vi "Periodic Tasks.vi"(8 "error in":errorcluster) -> ()   [LabVIEW 2012]
doc: "This VI runs in parallel to other tasks. It can contain as many user-defined periodic loops as you need. These can carry out PID or other sorts of timed response."
uses:
  <vilib>/Rock Robotics/WPI/Relay/WPI_RelayValue.ctl
  <vilib>/Rock Robotics/SystemInterfaces/Utilities/FPGA_UtilitiesLED Source.ctl
  <vilib>/Rock Robotics/SystemInterfaces/Utilities/FPGA_UtilitiesLED State.ctl
  <vilib>/Rock Robotics/WPI/Joystick/WPI_JoystickGetSetRefNum.vi
  Robot Global Data.vi
  <vilib>/Rock Robotics/WPI/Solenoid/WPI_SolenoidSetEnum.vi
  <vilib>/Rock Robotics/WPI/Compressor/WPI_CompressorGetSetRefNum.vi
panel:
  out "Ball Shooter motor speed":dbl
  out "s? t:f 4":dbl
  out "s? t:f 3":dbl
  out "s? t:f 2":dbl
  out "s? t:f":dbl
  out "Number of Balls in the Hopper":dbl
  in  "Starting Number Balls":i32=2
  out "Total Number of shots made":i16
  out "Hopper State":bool
  out "Ball in Hopper":bool
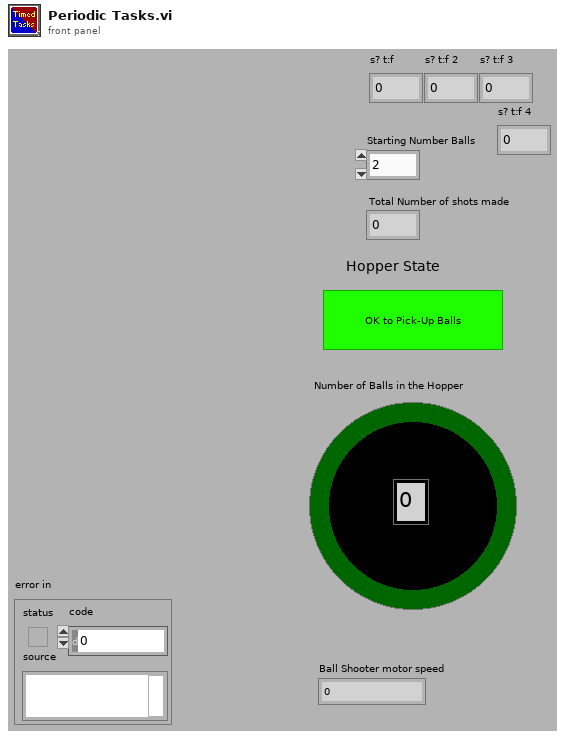
[diagram p1: front panel]
types:
  T1 = typedef "WPI_MotorControlDeviceRef.ctl" = cluster{"DeviceStatus":errorcluster, "Type":enum16{"PWM", "CAN"}, "PWM":cluster{"Digital Module":T2, "PWM Channel":T3, "DeadBand":T4}, "CAN":cluster{"Device Number":u8, "Control Mode":T5, "Semaphore":T6, "Max Vout":dbl}, "Invert":bool, "TransformRef":T7, "InvTransformRef":T7}
  T2 = typedef "FPGA_TypedefDigitalModule.ctl" = enum16{"Digital Module 1", "Digital Module 2"}
  T3 = typedef "FPGA_DIOPWMChannel.ctl" = enum8{"PWM 1", "PWM 2", "PWM 3", "PWM 4", "PWM 5", "PWM 6", "PWM 7", "PWM 8", "PWM 9", "PWM 10", "Invalid"}
  T4 = typedef "WPI_PWMDeadband.ctl" = cluster{"Name":string, "maxPositivePwm":i32, "minPositivePwm":i32, "centerPwm":i32, "maxNegativePwm":i32, "minNegativePwm":i32, "angularRange":u16}
  T5 = typedef "WPI_CANJaguar_ControlMode.ctl" = enum8{"Percent VBus", "Current", "Speed", "Position", "Voltage"}
  T6 = typedef "Semaphore RefNum" = refnum<k1>
  T7 = typedef "WPI_PWMTransform_ConPane.ctl" = refnum<vi>
  T8 = typedef "WPI_SolenoidDevRef.ctl" = cluster{"DevStatus":errorcluster, "Solenoid Module":T9, "Forward Solenoid Channel":T10, "Reverse Solenoid Channel":T10}
  T9 = typedef "FPGA_TypedefSolenoidModule.ctl" = enum16{"Solenoid Module 1", "Solenoid Module 2"}
  T10 = typedef "WPI_SolenoidChannel.ctl" = enum8{"Solenoid 1", "Solenoid 2", "Solenoid 3", "Solenoid 4", "Solenoid 5", "Solenoid 6", "Solenoid 7", "Solenoid 8", "Invalid"}
  T11 = typedef "WPI_JoystickDevRef.ctl" = cluster{"Device":T12}
  T12 = typedef "WPI_JoystickDeviceEnum.ctl" = enum16{"USB 1", "USB 2", "USB 3", "USB 4", "Kinect 1", "Kinect 2"}
  T13 = cluster{"MotorControlDevRef":T1, "MotorControlDevRef":T1, "MotorControlDevRef":T1, "MotorControlDevRef":T1}
  T14 = typedef "WPI_RelayValue.ctl" = enum16{"Off", "On", "Forward", "Reverse"}
  T15 = typedef "WPI_JoystickButtonState.ctl" = cluster{"Button 1":bool, "Button 2":bool, "Button 3":bool, "Button 4":bool, "Button 5":bool, "Button 6":bool, "Button 7":bool, "Button 8":bool, "Button 9":bool, "Button 10":bool, "Button 11":bool, "Button 12":bool}
  T16 = typedef "WPI_DigitalInputDevRef.ctl" = cluster{"DevStatus":errorcluster, "DIO Channel":T17, "Digital Module":T2}
  T17 = typedef "FPGA_DIOChannel.ctl" = enum8{"DIO 1", "DIO 2", "DIO 3", "DIO 4", "DIO 5", "DIO 6", "DIO 7", "DIO 8", "DIO 9", "DIO 10", "DIO 11", "DIO 12", "DIO 13", "DIO 14", "Invalid"}
  T18 = typedef "FPGA_UtilitiesLED State.ctl" = enum16{"Off", "On", "Toggle"}
  T19 = typedef "FPGA_UtilitiesLED Source.ctl" = enum16{"User LED", "FPGA LED"}
  T20 = typedef "WPI_CompressorDevRef.ctl" = cluster{"DevStatus":errorcluster, "DigitalInputDevRef":T16, "RelayDevRef":T21}
  T21 = typedef "WPI_RelayDevRef.ctl" = cluster{"DevStatus":errorcluster, "Relay Channel":T22, "Digital Module":T2, "Relay Direction":T23}
  T22 = typedef "FPGA_DIORelayChannel.ctl" = enum8{"Relay 1", "Relay 2", "Relay 3", "Relay 4", "Relay 5", "Relay 6", "Relay 7", "Relay 8", "Invalid"}
  T23 = typedef "WPI_RelayDirection.ctl" = enum16{"Both directions", "Forward only", "Reverse only"}
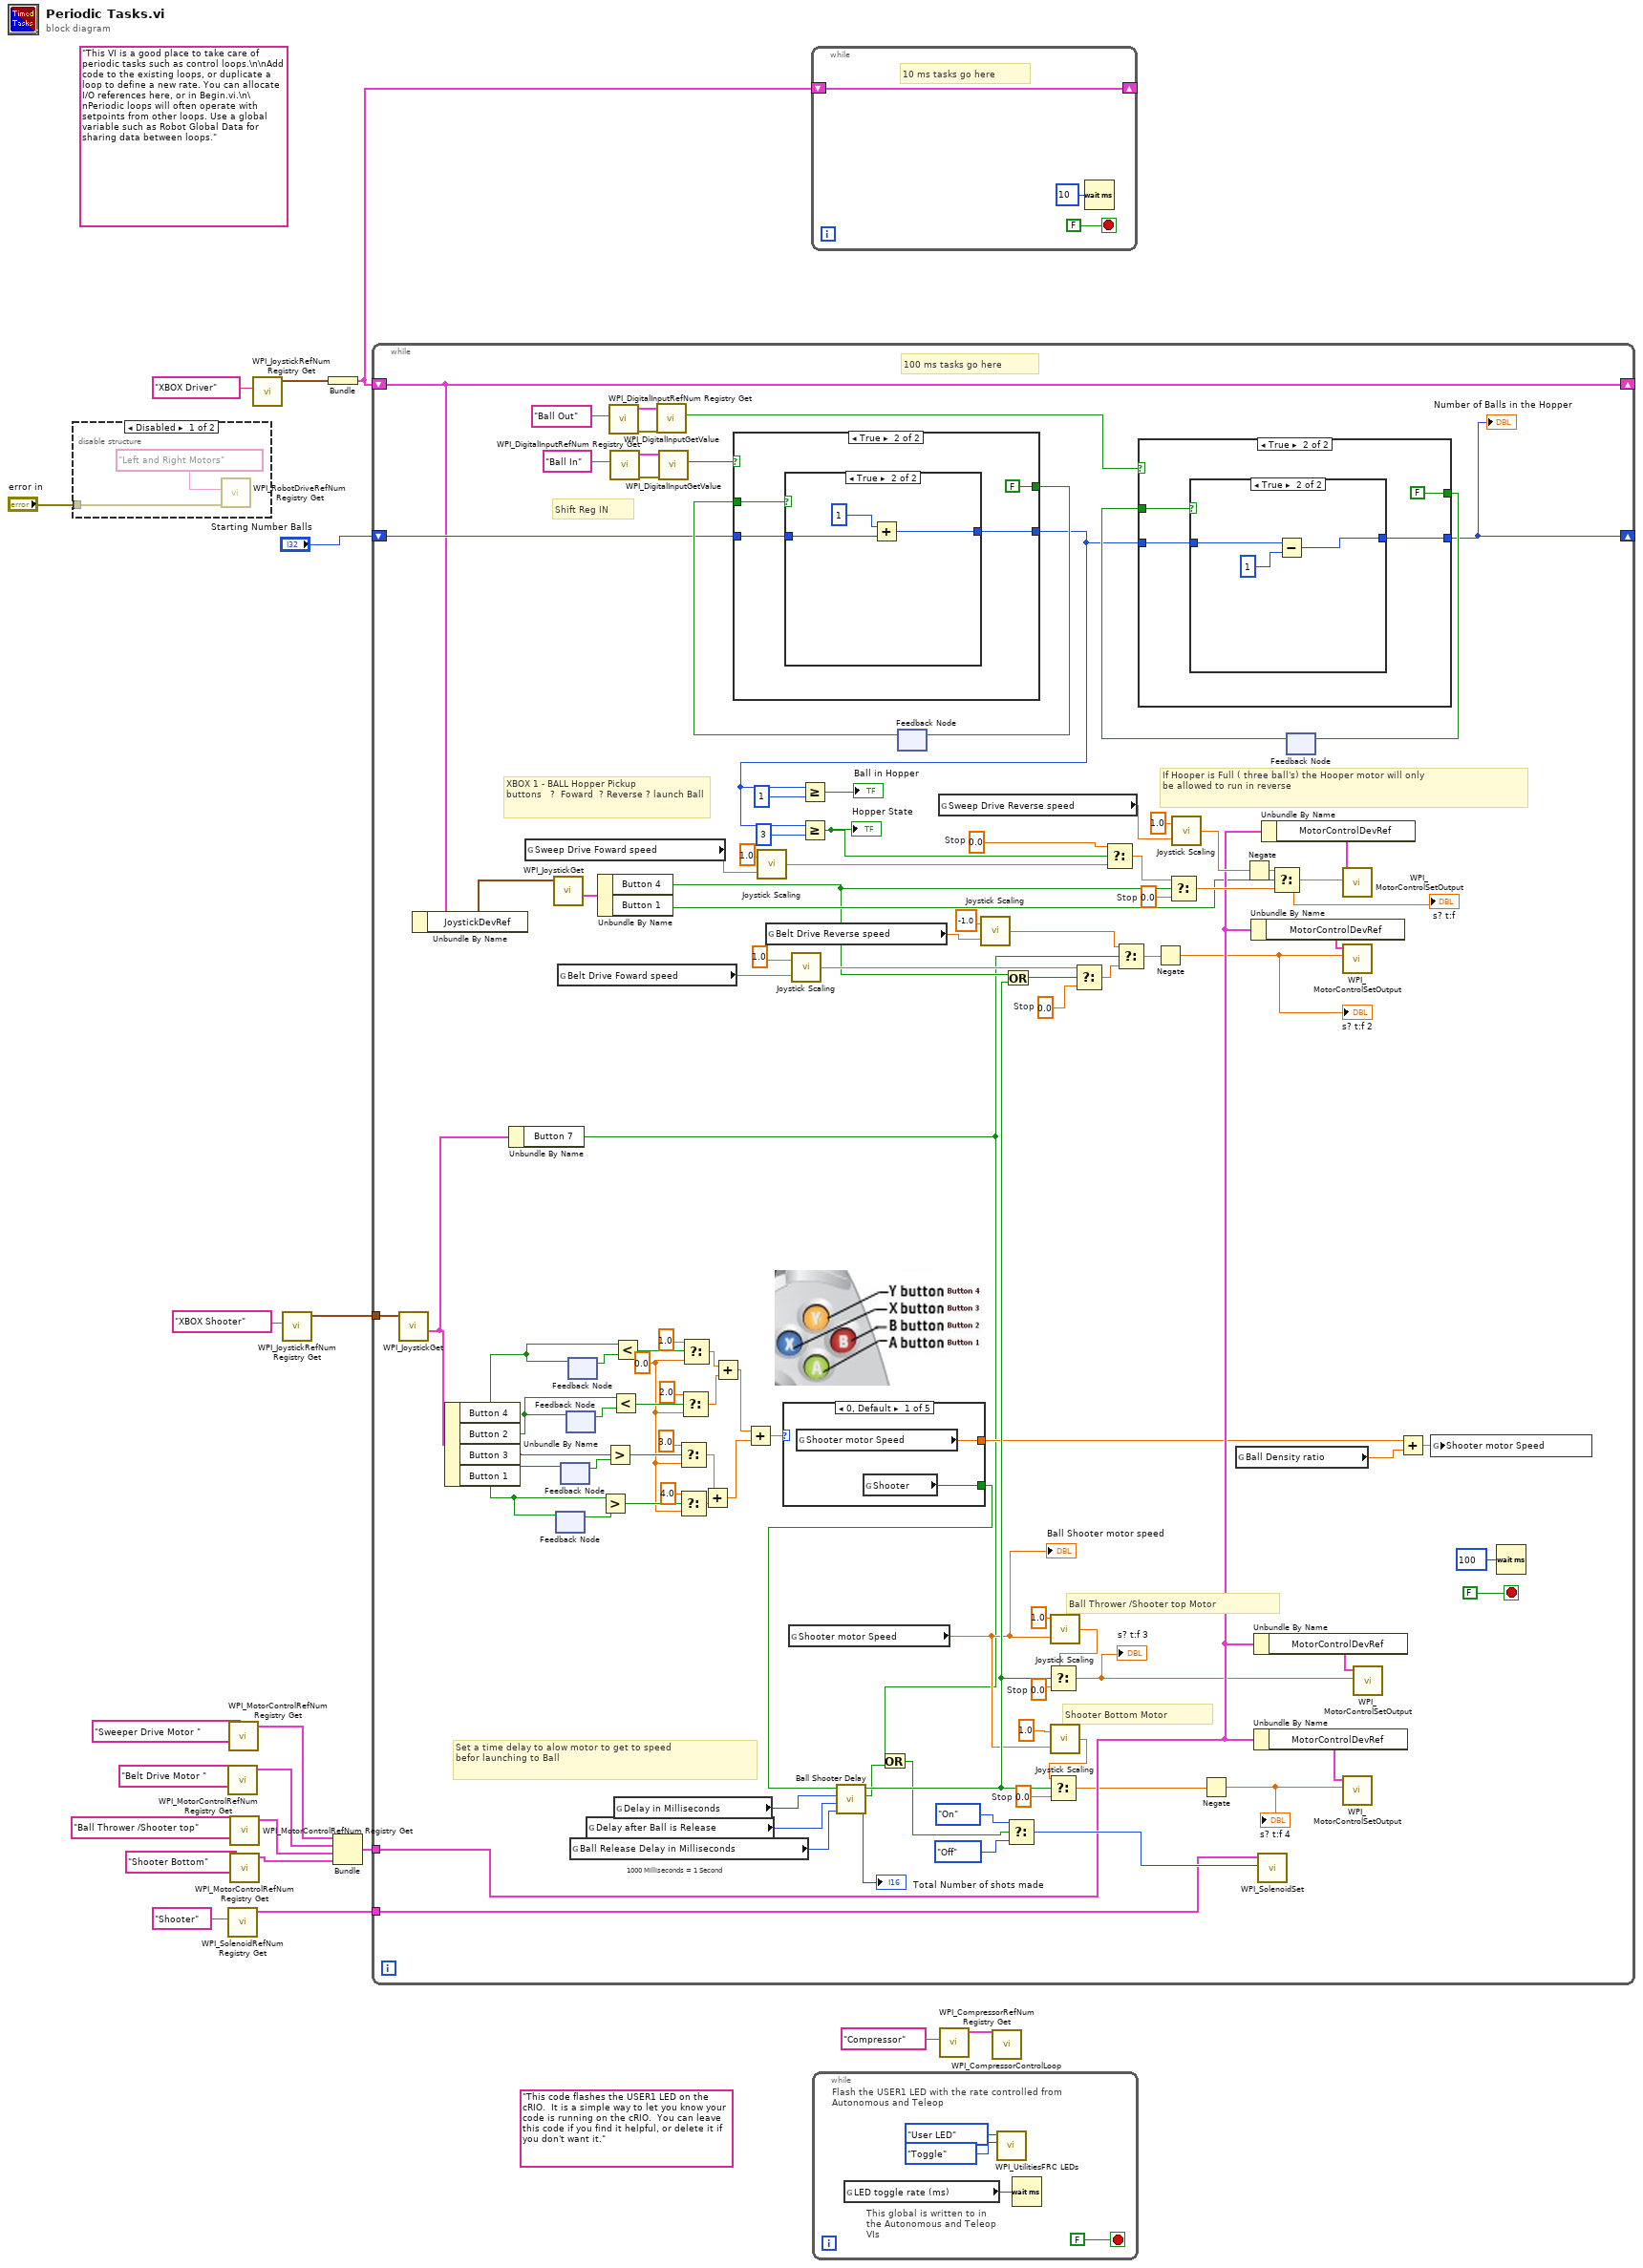
[diagram p0: block diagram]
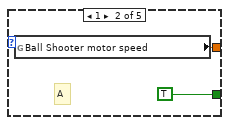
[diagram p3: hidden frame]
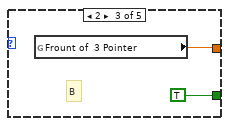
[diagram p4: hidden frame]
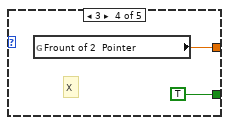
[diagram p5: hidden frame]
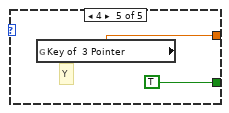
[diagram p6: hidden frame]
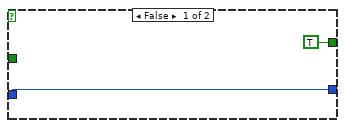
[diagram p7: hidden frame]
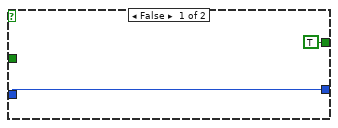
[diagram p9: hidden frame]
diagram:
  (unwired) "This code flashes the USER1 LED on the cRIO.  It is a simple way to let you know your code is running on the cRIO.  You can leave this code if you find it helpful, or delete it if you don't want it."
  (unwired) "This VI is a good place to take care of periodic tasks such as control loops.\n\nAdd code to the existing loops, or duplicate a loop to define a new rate. You can allocate I/O references here, or in Begin.vi.\n\nPeriodic loops will often operate with setpoints from other loops. Use a global variable such as Robot Global Data for sharing data between loops."
  n1 = disable-structure shown="Disabled" {
    disable-tunnel: "error in" -> [w21 _]
    frame Disabled {
      n2 = call <vilib>:"WPI_RobotDriveRefNum Registry Get.vi"("error in (no error)"=w21, "refnum name"="Left and Right Motors") -> ()  [unwired: 10 out]
    }
    frame Enabled {
    }
  }
  n3 = call <vilib>:"WPI_MotorControlRefNum Registry Get.vi"("refnum name"="Belt Drive Motor ") -> ("MotorControlDevRef"=w10:T1)  [unwired: 9 in, 1 out]
  n4 = call <vilib>:"WPI_SolenoidRefNum Registry Get.vi"("refnum name"="Shooter") -> ("SolenoidDevRef"=w4:T8)  [unwired: 9 in, 1 out]
  n5 = call <vilib>:"WPI_MotorControlRefNum Registry Get.vi"("refnum name"="Sweeper Drive Motor ") -> ("MotorControlDevRef"=w9:T1)  [unwired: 9 in, 1 out]
  n6 = call <vilib>:"WPI_MotorControlRefNum Registry Get.vi"("refnum name"="Ball Thrower /Shooter top") -> ("MotorControlDevRef"=w11:T1)  [unwired: 9 in, 1 out]
  n7 = call <vilib>:"WPI_MotorControlRefNum Registry Get.vi"("refnum name"="Shooter Bottom") -> ("MotorControlDevRef"=w7:T1)  [unwired: 9 in, 1 out]
  n8 = call <vilib>:"WPI_JoystickRefNum Registry Get.vi"("refnum name"="XBOX Driver") -> ("JoystickDevRef"=w20:T11)  [unwired: 1 in, 9 out]
  n9 = call <vilib>:"WPI_JoystickRefNum Registry Get.vi"("refnum name"="XBOX Shooter") -> ("JoystickDevRef"=w3:T11)  [unwired: 1 in, 9 out]
  n10 = Bundle("JoystickDevRef"=w20) -> (w19:cluster{"JoystickDevRef":T11})  [unwired: 1 out]
  n11 = Bundle("MotorControlDevRef"=w9, "MotorControlDevRef"=w10, "MotorControlDevRef"=w11, "MotorControlDevRef"=w7) -> (w12:T13)  [unwired: 1 out]
  n12 = while {
    shift-right: [w66] -> _
    shift-left: w19 -> [w66]
    shift-right: [w96] -> _
    shift-left: "Starting Number Balls" -> [w95]
    tunnel: w12 -> [w70]
    tunnel: w4 -> [w58]
    tunnel: w3 -> [w36]
    stop <- FALSE stop-if-true
    w41 = 0.0 ("t")
    w69 = 0.0  # Stop
    w106 = 0.0  # Stop
    w75 = 0.0  # Stop
    w109 = 0.0  # Stop
    w110 = 0.0  # Stop
    # "Ball Thrower /Shooter top Motor"
    # "Shooter Bottom Motor"
    # "Shift Reg IN"
    # "Set a time delay to alow motor to get to speed\nbefor launching to Ball"
    # "1000 Milliseconds = 1 Second"
    # "XBOX 1 - BALL Hopper Pickup\nbuttons   ?  Foward  ? Reverse ? launch Ball"
    # "If Hooper is Full ( three ball's) the Hooper motor will only\nbe allowed to run in reverse"
    # "100 ms tasks go here"
    n13 = call <vilib>:"WPI_JoystickGet.vi"("JoystickDevRef"=w36) -> ("Buttons"=w28:T15)  [unwired: 1 in, 5 out]
    n14 = Unbundle By Name(w66) -> ("JoystickDevRef"=w65:T11)
    n15 = Unbundle By Name(w28) -> ("Button 4"=w35:bool, "Button 2"=w34:bool, "Button 3"=w33:bool, "Button 1"=w32:bool)
    n16 = Unbundle By Name(w28) -> ("Button 7"=w25:bool)
    n17 = global read "Robot Global Data.vi" "Sweep Drive Foward speed"() -> (w82:dbl)
    n18 = call <vilib>:"WPI_JoystickGet.vi"("JoystickDevRef"=w65) -> ("Buttons"=w97:T15)  [unwired: 1 in, 5 out]
    n19 = feedback #1() -> (w53:bool)  [unwired: 1 in]
    n20 = feedback-in #1(w32) -> ()
    n21 = global read "Robot Global Data.vi" "Belt Drive Foward speed"() -> (w87:dbl)
    n22 = feedback #2() -> (w54:bool)  [unwired: 1 in]
    n23 = feedback-in #2(w33) -> ()
    n24 = feedback #3() -> (w55:bool)  [unwired: 1 in]
    n25 = feedback-in #3(w34) -> ()
    n26 = feedback #4() -> (w56:bool)  [unwired: 1 in]
    n27 = feedback-in #4(w35) -> ()
    n28 = global read "Robot Global Data.vi" "Ball Release Delay in Milliseconds"() -> (w101:i32)
    n29 = global read "Robot Global Data.vi" "Delay after Ball is Release"() -> (w100:u32)
    n30 = Unbundle By Name(w97) -> ("Button 4"=w67:bool, "Button 1"=w68:bool)
    n31 = Greater?(x=w32, y=w53) -> (0:w50:bool)
    n32 = Greater?(x=w33, y=w54) -> (0:w42:bool)
    n33 = call <vilib>:"WPI_DigitalInputRefNum Registry Get.vi"("refnum name"="Ball Out") -> ("error out"=w124:errorcluster, "DigitalInputDevRef"=w123:T16)  [unwired: 9 in]
    n34 = call <vilib>:"WPI_DigitalInputRefNum Registry Get.vi"("refnum name"="Ball In") -> ("error out"=w126:errorcluster, "DigitalInputDevRef"=w125:T16)  [unwired: 9 in]
    n35 = Less?(x=w34, y=w55) -> (x < y?=w51:bool)
    n36 = Less?(x=w35, y=w56) -> (x < y?=w52:bool)
    n37 = global read "Robot Global Data.vi" "Delay in Milliseconds"() -> (w99:i32)
    n38 = call <vilib>:"WPI_DigitalInputGetValue.vi"("error in (no error)"=w124, "DigitalInputDevRef"=w123) -> ("Value"=w113:bool)  [unwired: 7 in, 2 out]
    n39 = call <vilib>:"WPI_DigitalInputGetValue.vi"("error in (no error)"=w126, "DigitalInputDevRef"=w125) -> ("Value"=w114:bool)  [unwired: 7 in, 2 out]
    n40 = Select(t=3.0 ("f"), s=w42, f=w41) -> (s? t:f=w48:dbl)
    n41 = Select(t=4.0 ("f"), s=w50, f=w41) -> (s? t:f=w49:dbl)
    n42 = Select(t=2.0 ("f"), s=w51, f=w41) -> (s? t:f=w46:dbl)
    n43 = Select(t=1.0 ("f"), s=w52, f=w41) -> (s? t:f=w47:dbl)
    n44 = Add(x=w48, y=w49) -> (x+y=w45:dbl)
    n45 = Add(x=w47, y=w46) -> (x+y=w44:dbl)
    n46 = Add(x=w44, y=w45) -> (x+y=w43:dbl)
    n47 = call "Joystick Scaling.vi"("Scale (%)"=w82, "Input (+/- 1.00 volt)"=1.0) -> ("Output"=w81:dbl)  [unwired: 1 in]
    n48 = global read "Robot Global Data.vi" "Belt Drive Reverse speed"() -> (w85:dbl)
    n49 = case shown="0, Default" w43 {
      tunnel: [w130 TRUE TRUE TRUE TRUE] -> w31
      tunnel: [w129 w131 w133 w135 w137] -> w30
      frame 0, Default {
        n50 = global read "Robot Global Data.vi" "Shooter motor Speed"() -> (w129:dbl)
        n51 = global read "Robot Global Data.vi" "Shooter"() -> (w130:bool)
      }
      frame 1 {
        # "A"
        n52 = global read "Robot Global Data.vi" "Ball Shooter motor speed"() -> (w131:dbl)
      }
      frame 2 {
        # "B"
        n53 = global read "Robot Global Data.vi" "Frount of  3 Pointer"() -> (w133:dbl)
      }
      frame 3 {
        # "X"
        n54 = global read "Robot Global Data.vi" "Frount of 2  Pointer"() -> (w135:dbl)
      }
      frame 4 {
        # "Y"
        n55 = global read "Robot Global Data.vi" "Key of  3 Pointer"() -> (w137:dbl)
      }
    }
    n56 = global read "Robot Global Data.vi" "Shooter motor Speed"() -> (w29:dbl)
    "Ball Shooter motor speed" <- w29
    n57 = call "Joystick Scaling.vi"("Scale (%)"=w87, "Input (+/- 1.00 volt)"=1.0) -> ("Output"=w86:dbl)  [unwired: 1 in]
    n58 = call "Ball Shooter Delay.vi"("Ball Release \nDelay in Milliseconds"=w101, "Delay after Ball is Release"=w100, "Delay in Milliseconds"=w99, "Shoot ball"=w31) -> ("Total Number of shots made"=→"Total Number of shots made":i16, "Ball Release"=w26:bool, "Shooter Motor"=w71:bool)  [unwired: 5 in]
    n59 = Or(x=w25, y=w26) -> (x .or. y?=w27:bool)
    n60 = feedback #5() -> (w120:bool)  [unwired: 1 in]
    n61 = case shown="True" w114 {
      tunnel: w95 -> [w150 w154]
      tunnel: [w150 w153] -> w94
      tunnel: [TRUE FALSE] -> w119
      tunnel: w120 -> [_ w151]
      frame False {
      }
      frame True {
        n62 = case shown="True" w151 {
          tunnel: w154 -> [w155 w157]
          tunnel: [w155 w156] -> w153
          frame False {
          }
          frame True {
            n63 = Add(x=1, y=w157) -> (x+y=w156:i32)
          }
        }
      }
    }
    n64 = Greater Or Equal?(x=w94, y=1) -> (x >= y?=→"Ball in Hopper":bool)
    n65 = Greater Or Equal?(x=w94, y=3) -> (x >= y?=w112:bool)
    "Hopper State" <- w112
    n66 = feedback-in #5(w119) -> ()
    n67 = global read "Robot Global Data.vi" "Sweep Drive Reverse speed"() -> (w79:dbl)
    n68 = call "Joystick Scaling.vi"("Scale (%)"=w85, "Input (+/- 1.00 volt)"=-1.0) -> ("Output"=w84:dbl)  [unwired: 1 in]
    n69 = Or(x=w67, y=w71) -> (x .or. y?=w102:bool)
    n70 = Select(t=WPI_RelayValue."On" ("RelayValue"), s=w27, f=WPI_RelayValue."Off" ("RelayValue")) -> (s? t:f=w98:T14)
    n71 = call "Joystick Scaling.vi"("Scale (%)"=w29, "Input (+/- 1.00 volt)"=1.0) -> ("Output"=w73:dbl)  [unwired: 1 in]
    n72 = Select(t=w73, s=w71, f=w69) -> (s? t:f=w63:dbl)
    "s? t:f 3" <- w63
    n73 = call "Joystick Scaling.vi"("Scale (%)"=w29, "Input (+/- 1.00 volt)"=1.0) -> ("Output"=w90:dbl)  [unwired: 1 in]
    n74 = Select(t=w90, s=w71, f=w106) -> (s? t:f=w62:dbl)
    n75 = Select(t=w86, s=w102, f=w75) -> (s? t:f=w107:dbl)
    n76 = Select(t=w110, s=w112, f=w81) -> (s? t:f=w111:dbl)
    n77 = Select(t=w84, s=w25, f=w107) -> (s? t:f=w61:dbl)
    n78 = Negate(x=w61) -> (-x=w60:dbl)
    "s? t:f 2" <- w60
    n79 = Select(t=w111, s=w67, f=w109) -> (s? t:f=w108:dbl)
    n80 = call "Joystick Scaling.vi"("Scale (%)"=w79, "Input (+/- 1.00 volt)"=1.0) -> ("Output"=w80:dbl)  [unwired: 1 in]
    n81 = Negate(x=w62) -> (-x=w57:dbl)
    "s? t:f 4" <- w57
    n82 = global read "Robot Global Data.vi" "Ball Density ratio"() -> (w23:dbl)
    n83 = Negate(x=w80) -> (-x=w59:dbl)
    n84 = Unbundle By Name(w70) -> ("MotorControlDevRef"=w91:T1)
    n85 = Unbundle By Name(w70) -> ("MotorControlDevRef"=w72:T1)
    n86 = Unbundle By Name(w70) -> ("MotorControlDevRef"=w93:T1)
    n87 = call-poly <vilib>:"WPI_SolenoidSet.vi"("Value"=w98, "SolenoidDevRef"=w58) -> ()  [unwired: 8 in, 2 out]
    n88 = Unbundle By Name(w70) -> ("MotorControlDevRef"=w92:T1)
    n89 = Select(t=w59, s=w68, f=w108) -> (s? t:f=w64:dbl)
    "s? t:f" <- w64
    n90 = feedback #6() -> (w117:bool)  [unwired: 1 in]
    n91 = case shown="True" w113 {
      tunnel: w94 -> [w140 w144]
      tunnel: [w140 w143] -> w96
      tunnel: [TRUE FALSE] -> w118
      tunnel: w117 -> [_ w141]
      frame False {
      }
      frame True {
        n92 = case shown="True" w141 {
          tunnel: w144 -> [w145 w147]
          tunnel: [w145 w148] -> w143
          frame False {
          }
          frame True {
            n93 = Subtract(x=w147, y=1) -> (x-y=w148:i32)
          }
        }
      }
    }
    "Number of Balls in the Hopper" <- w96
    n94 = feedback-in #6(w118) -> ()
    n95 = call <vilib>:"WPI_MotorControlSetOutput.vi"("Output"=w64, "MotorControlDevRef"=w92) -> ()  [unwired: 7 in, 3 out]
    n96 = call <vilib>:"WPI_MotorControlSetOutput.vi"("Output"=w60, "MotorControlDevRef"=w91) -> ()  [unwired: 7 in, 3 out]
    n97 = call <vilib>:"WPI_MotorControlSetOutput.vi"("Output"=w57, "MotorControlDevRef"=w93) -> ()  [unwired: 7 in, 3 out]
    n98 = call <vilib>:"WPI_MotorControlSetOutput.vi"("Output"=w63, "MotorControlDevRef"=w72) -> ()  [unwired: 7 in, 3 out]
    n99 = Add(x=w30, y=w23) -> (x+y=w24:dbl)
    n100 = global write "Robot Global Data.vi" "Shooter motor Speed"(w24) -> ()
    n101 = Wait (ms)(milliseconds to wait=u32 100) -> ()  [unwired: 1 out]
  }
  n102 = while {
    shift-right: [w159] -> _
    shift-left: w19 -> [w159]
    stop <- FALSE stop-if-true
    # "10 ms tasks go here"
    n103 = Wait (ms)(milliseconds to wait=u32 10) -> ()  [unwired: 1 out]
  }
  n104 = while {
    stop <- FALSE stop-if-true
    # "This global is written to in the Autonomous and Teleop VIs"
    # "Flash the USER1 LED with the rate controlled from Autonomous and Teleop"
    n105 = global read "Robot Global Data.vi" "LED toggle rate (ms)"() -> (w162:u32)
    n106 = call <vilib>:"WPI_UtilitiesFRC LEDs.vi"("State"=FPGA_UtilitiesLED_State."Toggle", "LED Type"=FPGA_UtilitiesLED_Source."User LED") -> ()  [unwired: 1 in, 9 out]
    n107 = Wait (ms)(milliseconds to wait=w162) -> ()  [unwired: 1 out]
  }
  n108 = call <vilib>:"WPI_CompressorRefNum Registry Get.vi"("refnum name"="Compressor") -> ("CompressorDevRef"=w17:T20)  [unwired: 9 in, 1 out]
  n109 = call <vilib>:"WPI_CompressorControlLoop.vi"("CompressorDevRef"=w17) -> ()  [unwired: 11 in]
